vi "emi_Time Diff Monitoring.vi"(5 "Previous Time":u32, 9 "error in (no error)":errorcluster) -> (6 "Current Time":u32, 8 "Time Difference(ms)":u32, 10 "error out":errorcluster)   [LabVIEW 2011]
doc: "Use this to se the number of ms an action takes. They need be chained together for full effect.\n\nOn Error in. No change in behavior"
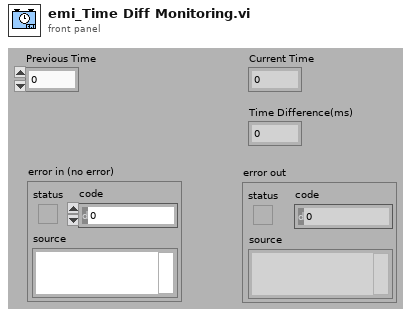
[diagram p1: front panel]
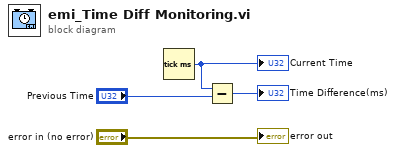
[diagram p0: block diagram]
diagram:
  n1 = Tick Count (ms)() -> (millisecond timer value=w4:u32)
  "Current Time" <- w4
  n2 = Subtract(x=w4, y="Previous Time") -> (x-y=→"Time Difference(ms)":u32)
  "error out" <- "error in (no error)"
